vi "Current Step.vi"(8 "error in (no error)":errorcluster, 11 "Double Scanner in":refnum<class "Double Scanner.lvclass">) -> (0 "error out":errorcluster, 1 "Total steps":i32, 2 "Current step":u32, 3 "Double Scanner out":refnum<class "Double Scanner.lvclass">)   [LabVIEW 2012, in "Double Scanner.lvclass"]
uses:
  Double Scanner.lvclass
  Scanner/Scanner.lvclass
panel:
  out "Ind Vars[i]":dbl
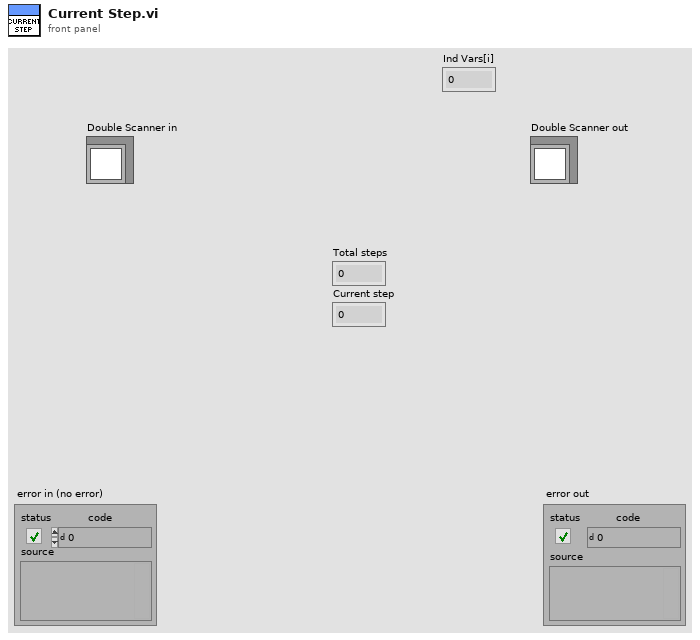
[diagram p1: front panel]
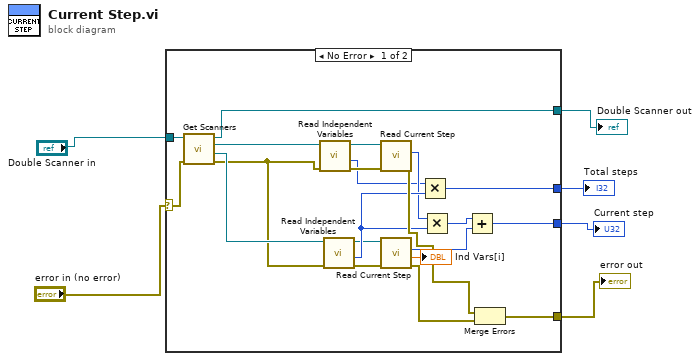
[diagram p0: block diagram]
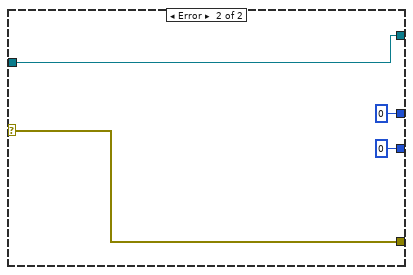
[diagram p2: hidden frame]
diagram:
  n1 = case shown="No Error" "error in (no error)" {
    selector: "error in (no error)" -> [w13 w31]
    tunnel: "Double Scanner in" -> [w14 w30]
    tunnel: [w11 w31] -> w4
    tunnel: [w10 0] -> w3
    tunnel: [w9 u32 0] -> w2
    tunnel: [w8 w30] -> w1
    frame No Error {
      n2 = call-dynamic "Get Scanners.vi"("error in (no error)"=w13, "Double Scanner in"=w14) -> ("error out"=w12:errorcluster, "Scanner 2 out"=w26:refnum<class "Scanner.lvclass">, "Scanner 1 out"=w27:refnum<class "Scanner.lvclass">, "Double Scanner out"=w8:refnum<class "Double Scanner.lvclass">)  [unwired: 6 in]
      n3 = call-dynamic "Read Independent Variables.vi"("error in (no error)"=w12, "Scanner.lvclass in"=w27) -> ("error out"=w21:errorcluster, "size"=w17:i32, "Scanner.lvclass out"=w16:refnum<class "Scanner.lvclass">)  [unwired: 4 in, 3 out]
      n4 = call-dynamic "Read Independent Variables.vi"("error in (no error)"=w12, "Scanner.lvclass in"=w26) -> ("error out"=w20:errorcluster, "size"=w19:i32, "Scanner.lvclass out"=w15:refnum<class "Scanner.lvclass">)  [unwired: 4 in, 3 out]
      n5 = call-dynamic "Read Current Step.vi"("error in (no error)"=w21, "Scanner.lvclass in"=w16) -> ("error out"=w24:errorcluster, "Current Step"=w18:u32)  [unwired: 6 in, 2 out]
      n6 = call-dynamic "Read Current Step.vi"("error in (no error)"=w20, "Scanner.lvclass in"=w15) -> ("error out"=w25:errorcluster, "Current Position"=→"Ind Vars[i]":dbl, "Current Step"=w22:u32)  [unwired: 6 in, 1 out]
      n7 = Multiply(x=w17, y=w19) -> (x*y=w10:i32)
      n8 = Multiply(x=w18, y=w19) -> (x*y=w23:u32)
      n9 = Add(x=w23, y=w22) -> (x+y=w9:u32)
      n10 = Merge Errors(w24, w25) -> (w11:errorcluster)
    }
    frame Error {
    }
  }
  "Total steps" <- w3
  "Current step" <- w2
  "error out" <- w4
  "Double Scanner out" <- w1
